vi "SwerveFieldCentric (SubVI).vi"(8 "Gyro Angle (deg)":dbl, 9 "Y":dbl, 11 "X":dbl) -> (1 "X*":dbl, 3 "Y*":dbl)   [LabVIEW 2020]
panel:
  out "X*Normalized":dbl
  out "Y* Normalized":dbl
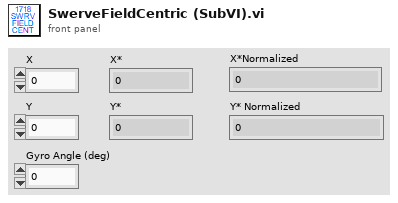
[diagram p1: front panel]
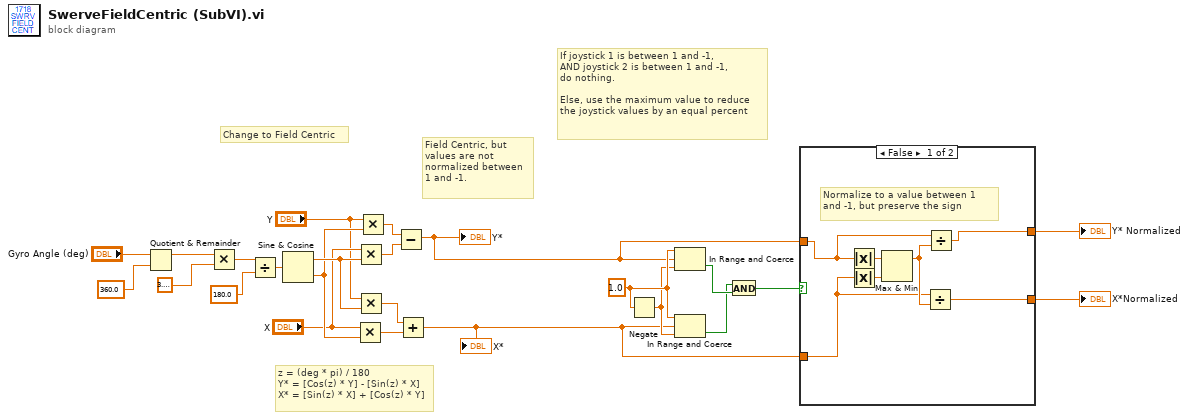
[diagram p0: block diagram]
diagram:
  w14 = 1.0 ("upper limit")
  # "z = (deg * pi) / 180\nY* = [Cos(z) * Y] - [Sin(z) * X]\nX* = [Sin(z) * X] + [Cos(z) * Y]"
  # "Field Centric, but\nvalues are not\nnormalized between\n1 and -1."
  # "Change to Field Centric"
  # "If joystick 1 is between 1 and -1,\nAND joystick 2 is between 1 and -1,\ndo nothing.\n\nElse, use the maximum value to reduce\nthe joystick values by an equal percent"
  n1 = Quotient & Remainder(x="Gyro Angle (deg)", y=360.0) -> (x-y*floor(x/y)=w1:dbl)  [unwired: 1 out]
  n2 = Multiply(x=w1, y=3.141592653589793) -> (x*y=w15:dbl)
  n3 = Divide(x=w15, y=180.0) -> (x/y=w16:dbl)
  n4 = Sine & Cosine(0:w16) -> (1:w18:dbl, 2:w17:dbl)
  n5 = Multiply(x="X", y=w17) -> (x*y=w23:dbl)
  n6 = Multiply(x="X", y=w18) -> (x*y=w21:dbl)
  n7 = Multiply(x="Y", y=w18) -> (x*y=w24:dbl)
  n8 = Multiply(x="Y", y=w17) -> (x*y=w22:dbl)
  n9 = Subtract(x=w22, y=w21) -> (x-y=w9:dbl)
  "Y*" <- w9
  n10 = Add(x=w24, y=w23) -> (x+y=w8:dbl)
  "X*" <- w8
  n11 = Negate(x=w14) -> (-x=w13:dbl)
  n12 = In Range and Coerce(upper limit=w14, x=w9, lower limit=w13) -> (In Range?=w12:bool)  [unwired: 1 out]
  n13 = In Range and Coerce(upper limit=w14, x=w8, lower limit=w13) -> (In Range?=w11:bool)  [unwired: 1 out]
  n14 = And(x=w11, y=w12) -> (x .and. y?=w10:bool)
  n15 = case shown="False" w10 {
    tunnel: [w26 w33] -> w7
    tunnel: w9 -> [w30 w33]
    tunnel: [w25 w32] -> w6
    tunnel: w8 -> [w28 w32]
    frame False {
      # "Normalize to a value between 1 and -1, but preserve the sign"
      n16 = Absolute Value(x=w30) -> (abs(x)=w29:dbl)
      n17 = Absolute Value(x=w28) -> (abs(x)=w27:dbl)
      n18 = Max & Min(x=w29, y=w27) -> (max(x,y)=w31:dbl)  [unwired: 1 out]
      n19 = Divide(x=w28, y=w31) -> (x/y=w25:dbl)
      n20 = Divide(x=w30, y=w31) -> (x/y=w26:dbl)
    }
    frame True {
    }
  }
  "Y* Normalized" <- w7
  "X*Normalized" <- w6
